vi "2048_main(login).vi"() -> ()   [LabVIEW 2021]
panel:
  out "String":string
  in  "OK Button":bool
  in  "密碼":string
  in  "帳號":string
  # "帳號:Labview\n密碼:123"
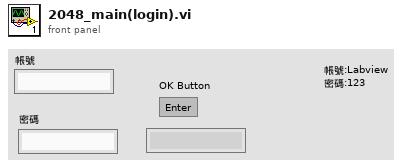
[diagram p1: front panel]
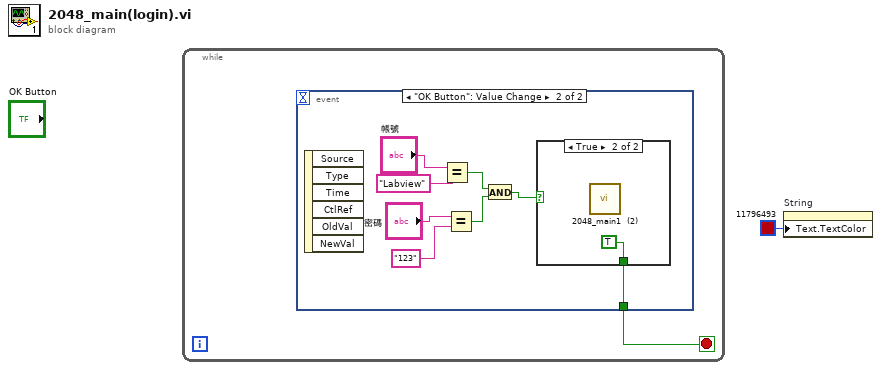
[diagram p0: block diagram]
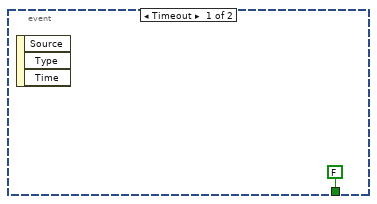
[diagram p2: hidden frame]
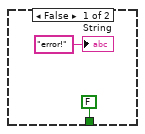
[diagram p3: hidden frame]
diagram:
  n1 = while {
    stop <- w2 stop-if-true
    n2 = event shown="[1] \"OK Button\": Value Change" {
      selector: _ -> [_ _]
      dyn-events: _ -> [_ _]
      timeout: _ -> [_ _]
      tunnel: [FALSE w4] -> w2
      event Timeout {
        n3 = event-data() -> ()  [unwired: 1 in, 3 out]
      }
      event "OK Button": Value Change {
        n4 = event-data() -> ()  [unwired: 1 in, 6 out]
        n5 = Equal?(x="帳號", y="Labview") -> (x = y?=w7:bool)
        n6 = Equal?(x="密碼", y="123") -> (x = y?=w6:bool)
        n7 = And(x=w7, y=w6) -> (x .and. y?=w5:bool)
        n8 = case shown="True" w5 {
          tunnel: [FALSE TRUE] -> w4
          frame False {
            "String" <- "error!" ("String")
          }
          frame True {
            n9 = call "2048_main1  (2).vi"() -> ()  [unwired: 12 in]
          }
        }
      }
    }
  }
  n10 = property on="String" class="Str"("Text.TextColor"=u32 11796493 ("Text.Text Colors:Text Color")) -> ()  [unwired: 2 in, 2 out]
